vi "get autostart enable status.vi"(8 "error in (no error)":errorcluster, 11 "Cobolt in":refnum<class "Cobolt.lvclass">) -> (0 "error out":errorcluster, 3 "Cobolt out":refnum<class "Cobolt.lvclass">)   [LabVIEW 2012, in "Cobolt.lvclass"]
uses:
  Cobolt.lvclass
  CoboltLaserDrivers_Public_LV2012/CoboltLaser_Controls/ExpectedResponseType.ctl
  Cobolt.lvclass/Cobolt.ctl
panel:
  out "buffer out":string
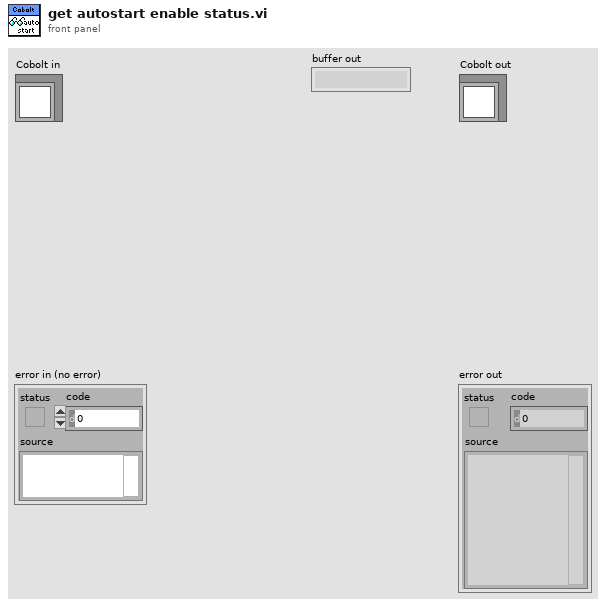
[diagram p1: front panel]
types:
  T1 = typedef "Cobolt.lvclass/ExpectedResponseType.ctl" = u16
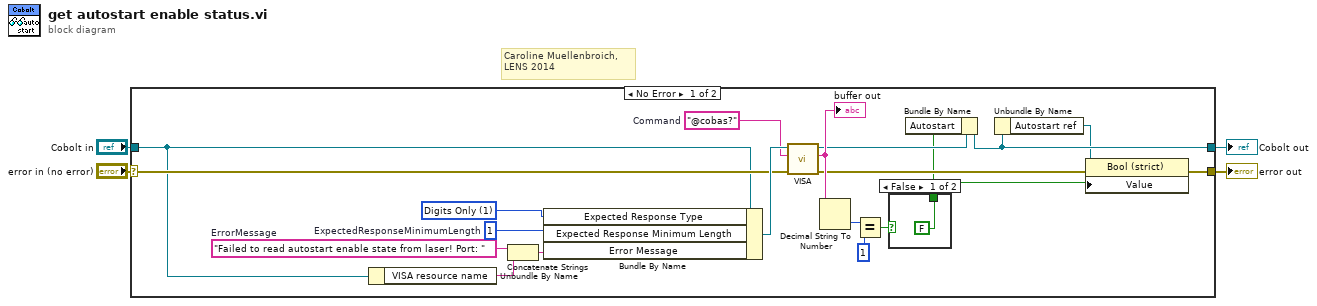
[diagram p0: block diagram]
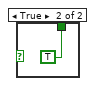
[diagram p2: hidden frame]
diagram:
  # "Caroline Muellenbroich, \nLENS 2014"
  n1 = case shown="No Error" "error in (no error)" {
    selector: "error in (no error)" -> [w11 w27]
    tunnel: [w7 w27] -> w3
    tunnel: [w9 w26] -> w1
    tunnel: "Cobolt in" -> [w10 w26]
    frame No Error {
      w19 = T1 1 items=["Any", "Digits Only", "Non-Digits Only"] ("ExpectedResponseType")
      w15 = 1  # ExpectedResponseMinimumLength
      w17 = "Failed to read autostart enable state from laser! Port: "  # ErrorMessage
      w13 = "@cobas?"  # Command
      n2 = Unbundle By Name(w10) -> ("VISA resource name"=w16:string)
      n3 = Concatenate Strings(w17, w16) -> (w18:string)
      n4 = Bundle By Name(cluster=w10, "Expected Response Type"=w19, "Expected Response Minimum Length"=w15, "Error Message"=w18) -> (w14:refnum<class "Cobolt.lvclass">)
      n5 = call-dynamic "VISA.vi"("error in (no error)"=w11, "string to write"=w13, "Cobolt in"=w14) -> ("error out"=w8:errorcluster, "buffer out"=w22:string, "Cobolt out"=w12:refnum<class "Cobolt.lvclass">)  [unwired: 6 in]
      "buffer out" <- w22
      n6 = Decimal String To Number(string=w22) -> (number=w21:i32)  [unwired: 2 in, 1 out]
      n7 = Equal?(x=w21, y=1) -> (x = y?=w23:bool)
      n8 = case shown="False" w23 {
        tunnel: [FALSE TRUE] -> w5
        frame False {
        }
        frame True {
        }
      }
      n9 = Bundle By Name(cluster=w12, "Autostart"=w5) -> (w9:refnum<class "Cobolt.lvclass">)
      n10 = Unbundle By Name(w9) -> ("Autostart ref"=w6:refnum<vi>)
      n11 = property class="Bool (strict)"(reference=w6, error in=w8, "Value"=w5) -> (error out=w7:errorcluster)  [unwired: 1 out]
    }
    frame Error {
    }
  }
  "error out" <- w3
  "Cobolt out" <- w1
